vi "niFpgaRegisterEmulation.vi"(0 "name":string, 1 "in timed loop":bool, 5 "Initial Value":variant[](array[variant]), 7 "data in":i32, 9 "write":bool, 11 "error in (no error)":errorcluster, 12 "Local? (F)":bool, 13 "Ref In wired (F)":bool) -> (8 "data out":i32, 15 "error out":errorcluster)   [LabVIEW 2017]
uses:
  <instcachedir>/0/niFpgaRegisterEmulationFpgaImpl_443A04883B3343BC9BF1EB853D0E50EA.lvgen/niFpgaRegisterEmulationFpgaImpl_443A04883B3343BC9BF1EB853D0E50EA_000.vi
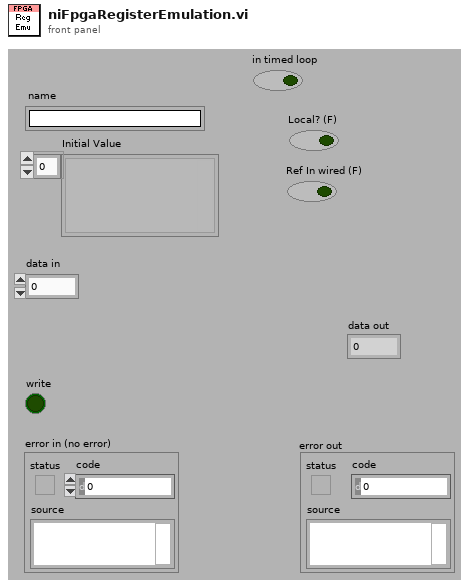
[diagram p1: front panel]
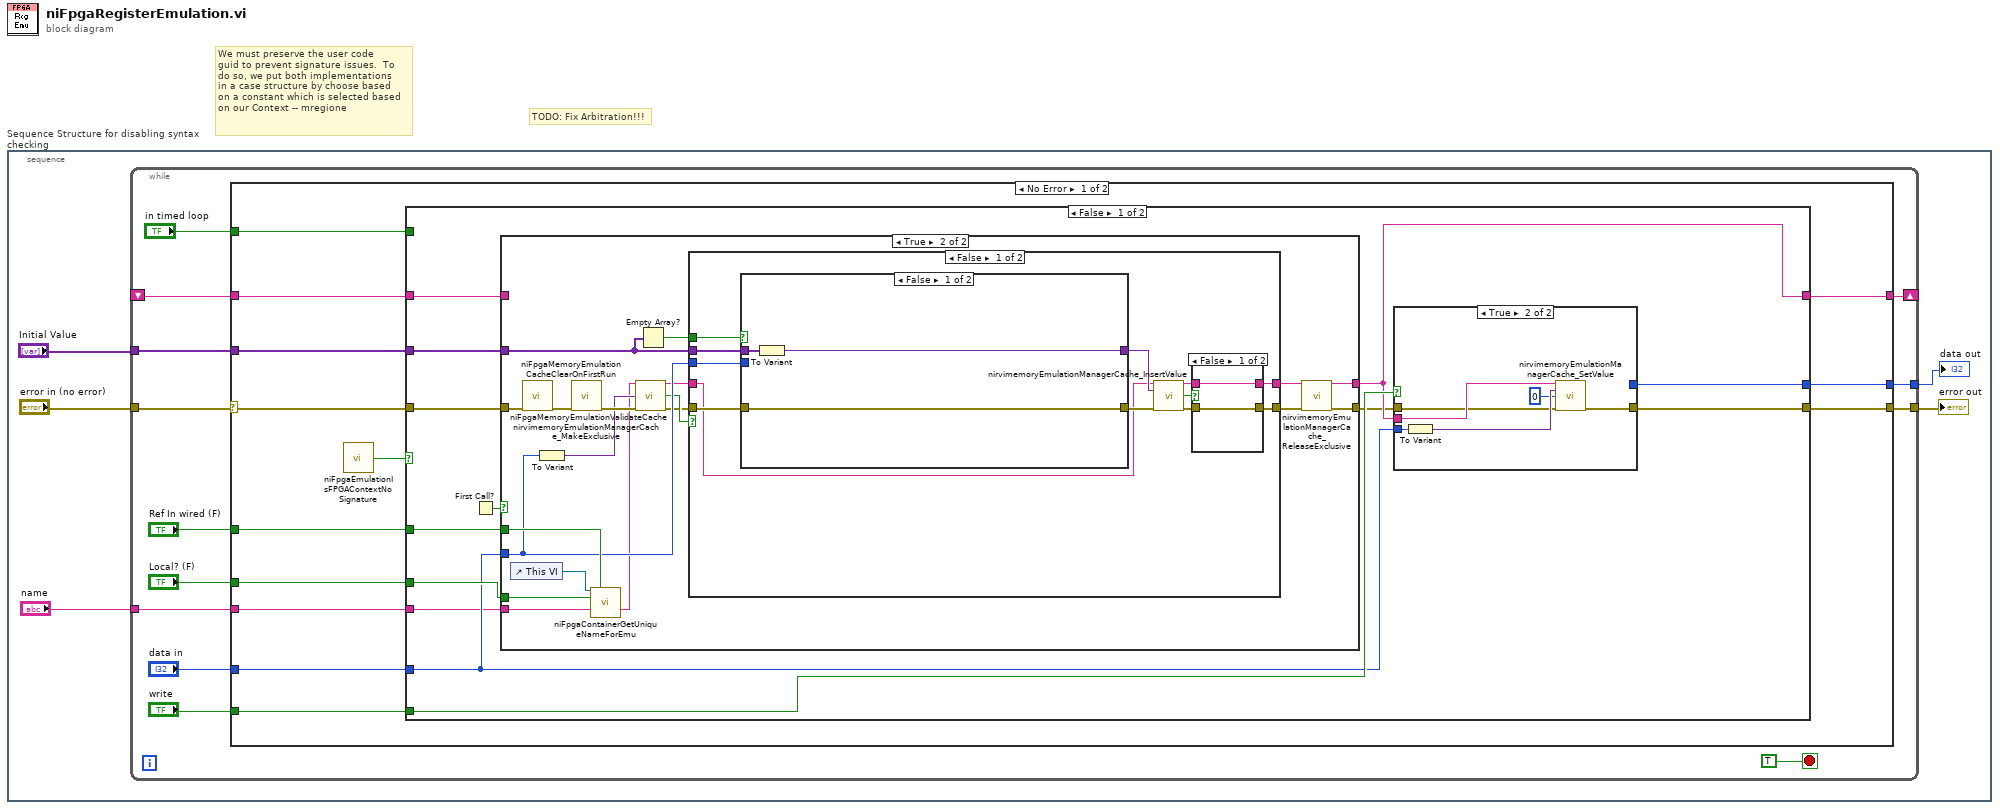
[diagram p0: block diagram]
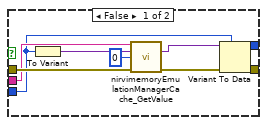
[diagram p2: hidden frame]
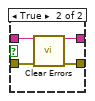
[diagram p4: hidden frame]
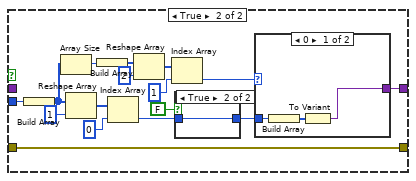
[diagram p5: hidden frame]
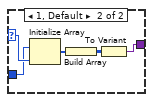
[diagram p6: hidden frame]
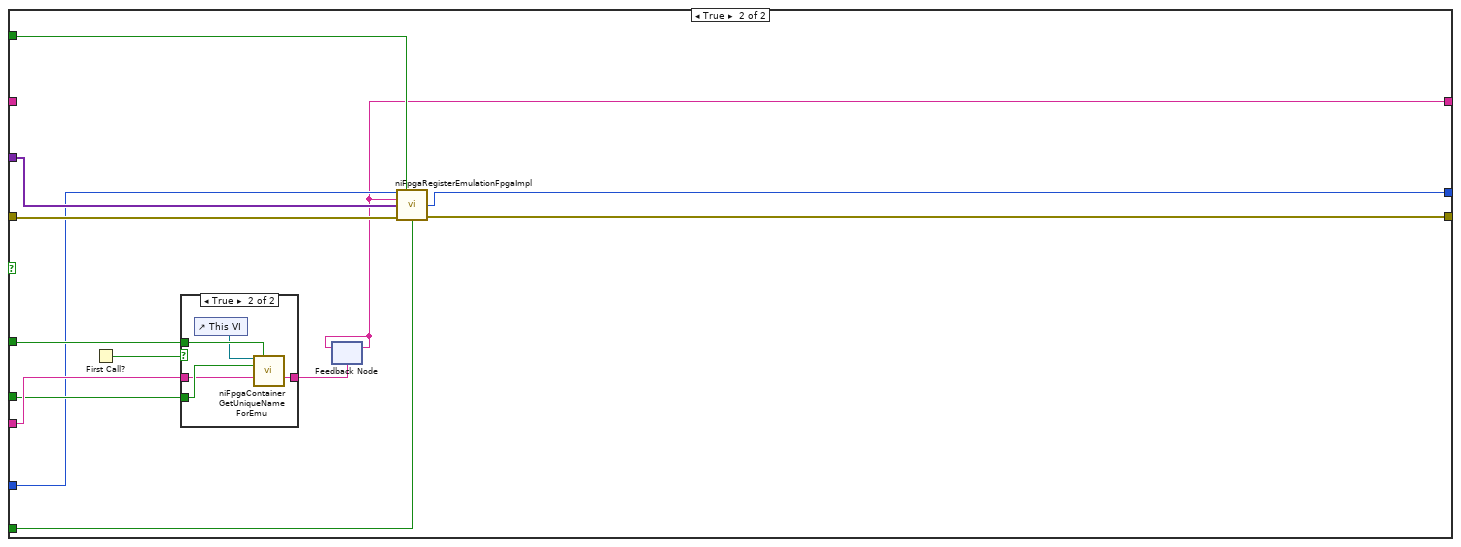
[diagram p9: hidden frame]
diagram:
  # "We must preserve the user code\nguid to prevent signature issues.  To\ndo so, we put both implementations\nin a case structure by choose based\non a constant which is selected based\non our Context -- mregione"
  # "TODO: Fix Arbitration!!!"
  n1 = stacked-sequence "Sequence Structure for disabling syntax checking" {
    frame #0 {
      n2 = while {
        tunnel: [w17] -> w5
        tunnel: "error in (no error)" -> [w15]
        tunnel: "Initial Value" -> [w11]
        shift-right: [w8] -> _
        shift-left: _ -> [w9]
        tunnel: [w7] -> w3
        tunnel: "name" -> [w6]
        stop <- TRUE stop-if-true
        n3 = case shown="No Error" w15 {
          selector: w15 -> [w31 w148]
          tunnel: w11 -> [w28 _]
          tunnel: [w25 w148] -> w17
          tunnel: "data in" -> [w23 w146]
          tunnel: "write" -> [w27 _]
          tunnel: "Ref In wired (F)" -> [w30 _]
          tunnel: "Local? (F)" -> [w29 _]
          tunnel: "in timed loop" -> [w26 _]
          tunnel: w9 -> [w21 w147]
          tunnel: [w20 w147] -> w8
          tunnel: [w24 w146] -> w7
          tunnel: w6 -> [w22 _]
          frame No Error {
            n4 = call <vilib>:"niFpgaEmulationIsFPGAContextNoSignature.vi"() -> ("Is Fpga Context?"=w19:bool)  [unwired: 15 in]
            n5 = case shown="False" w19 {
              tunnel: w31 -> [w44 w134]
              tunnel: w30 -> [w43 w135]
              tunnel: w29 -> [w42 w136]
              tunnel: w28 -> [w41 w132]
              tunnel: w27 -> [w40 w133]
              tunnel: w26 -> [_ w138]
              tunnel: [w39 w128] -> w25
              tunnel: [w38 w129] -> w24
              tunnel: w23 -> [w37 w131]
              tunnel: w22 -> [w36 w137]
              tunnel: w21 -> [w35 _]
              tunnel: [w34 w130] -> w20
              frame False {
                n6 = First Call?() -> (First Call?: T/F=w32:bool)
                n7 = case shown="True" w32 {
                  tunnel: [w61 w64] -> w33
                  tunnel: w44 -> [w61 w63]
                  tunnel: w41 -> [_ w79]
                  tunnel: w37 -> [_ w73]
                  tunnel: w43 -> [_ w77]
                  tunnel: w42 -> [_ w76]
                  tunnel: w36 -> [_ w75]
                  tunnel: [w60 w65] -> w34
                  tunnel: w35 -> [w60 _]
                  frame False {
                  }
                  frame True {
                    n8 = control-ref of="This VI"() -> (w78:refnum<vi>)
                    n9 = call <vilib>:"niFpgaMemoryEmulationCacheClearOnFirstRun.vi"("error in"=w63) -> ("error out"=w62:errorcluster)  [unwired: 13 in, 1 out]
                    n10 = To Variant(anything=w73) -> (Variant=w72:variant)
                    n11 = call <vilib>:"nirvimemoryEmulationManagerCache_MakeExclusive.vi"("error in"=w62) -> ("error out"=w74:errorcluster)  [unwired: 13 in, 1 out]
                    n12 = call <vilib>:"niFpgaContainerGetUniqueNameForEmu.vi"("parent VI"=w78, "ref in wired"=w77, "local"=w76, "name in"=w75) -> ("name out"=w71:string)  [unwired: 11 in]
                    n13 = call <vilib>:"niFpgaMemoryEmulationValidateCache.vi"("key"=w71, "Data In"=w72, "error in"=w74) -> ("key (dup)"=w68:string, "found?"=w70:bool, "error out"=w69:errorcluster)  [unwired: 10 in]
                    n14 = Empty Array?(array=w79) -> (empty?=w80:bool)
                    n15 = case shown="False" w70 {
                      tunnel: w80 -> [w92 _]
                      tunnel: w79 -> [w91 _]
                      tunnel: [w86 w127] -> w67
                      tunnel: w73 -> [w84 _]
                      tunnel: w69 -> [w83 w127]
                      tunnel: w68 -> [w82 w126]
                      tunnel: [w81 w126] -> w66
                      frame False {
                        n16 = case shown="False" w92 {
                          tunnel: w91 -> [w100 _]
                          tunnel: [w99 w102] -> w90
                          tunnel: w84 -> [_ w116]
                          tunnel: w83 -> [w98 w101]
                          tunnel: [w98 w101] -> w87
                          frame False {
                            n17 = To Variant(anything=w100) -> (Variant=w99:variant)
                          }
                          frame True {
                            n18 = Build Array(w116) -> (w115:i32[])
                            n19 = Array Size(array=w115) -> (size(s)=w111:i32)
                            n20 = Reshape Array(w115, 1 ("dimension size")) -> (w113:i32[])
                            n21 = Build Array(w111) -> (w107:i32[])
                            n22 = Index Array(array=w113, index=0) -> (element=w106:i32)
                            n23 = Reshape Array(w107, 2 ("dimension size")) -> (w108:i32[])
                            n24 = Index Array(array=w108, index=1) -> (element=w104:i32)
                            n25 = case shown="True" FALSE {
                              tunnel: w106 -> [_ w125]
                              tunnel: [_ w125] -> w103
                              frame False {
                              }
                              frame True {
                              }
                            }
                            n26 = case shown="0" w104 {
                              selector: w104 -> [_ w124]
                              tunnel: w103 -> [w119 w123]
                              tunnel: [w117 w120] -> w102
                              frame 0 {
                                n27 = Build Array(w119) -> (w118:i32[])
                                n28 = To Variant(anything=w118) -> (Variant=w117:variant)
                              }
                              frame 1, Default {
                                n29 = Initialize Array(w123, w124) -> (w122:i32[])
                                n30 = Build Array(w122) -> (w121:i32[][])
                                n31 = To Variant(anything=w121) -> (Variant=w120:variant)
                              }
                            }
                          }
                        }
                        n32 = call <vilib>:"nirvimemoryEmulationManagerCache_InsertValue.vi"("Key"=w82, "Value"=w90, "error in (no error)"=w87) -> ("Key"=w85:string, "Found"=w89:bool, "error out"=w88:errorcluster)  [unwired: 1 in, 9 out]
                        n33 = case shown="False" w89 {
                          tunnel: w88 -> [w94 w96]
                          tunnel: [w94 w95] -> w86
                          tunnel: [w93 w97] -> w81
                          tunnel: w85 -> [w93 w97]
                          frame False {
                          }
                          frame True {
                            n34 = call <vilib>:"Clear Errors.vi"("error in (no error)"=w96) -> ("error out"=w95:errorcluster)  [unwired: 1 in, 5 out]
                          }
                        }
                      }
                      frame True {
                      }
                    }
                    n35 = call <vilib>:"nirvimemoryEmulationManagerCache_ReleaseExclusive.vi"("Key"=w66, "error in"=w67) -> ("Key (dup)"=w65:string, "error out"=w64:errorcluster)  [unwired: 12 in]
                  }
                }
                n36 = case shown="True" w40 {
                  tunnel: w37 -> [w46 w59]
                  tunnel: w33 -> [w51 w56]
                  tunnel: w34 -> [w50 w57]
                  tunnel: [w48 w55] -> w39
                  tunnel: [w47 _] -> w38
                  frame False {
                    n37 = To Variant(anything=w46) -> (Variant=w53:variant)
                    n38 = call <vilib>:"nirvimemoryEmulationManagerCache_GetValue.vi"("Key"=w50, "Value"=w53, "Address"=0, "error in (no error)"=w51) -> ("Value"=w45:variant, "error out"=w49:errorcluster)  [unwired: 10 out]
                    n39 = Variant To Data(error in=w49, type=w46, Variant=w45) -> (data=w47:i32, error out=w48:errorcluster)
                  }
                  frame True {
                    n40 = To Variant(anything=w59) -> (Variant=w58:variant)
                    n41 = call <vilib>:"nirvimemoryEmulationManagerCache_SetValue.vi"("Key"=w57, "Value"=w58, "Address"=0, "error in (no error)"=w56) -> ("error out"=w55:errorcluster)  [unwired: 11 out]
                  }
                }
              }
              frame True {
                n42 = First Call?() -> (First Call?: T/F=w140:bool)
                n43 = case shown="True" w140 {
                  tunnel: w136 -> [_ w145]
                  tunnel: w135 -> [_ w144]
                  tunnel: [_ w142] -> w139
                  tunnel: w137 -> [_ w141]
                  frame False {
                  }
                  frame True {
                    n44 = control-ref of="This VI"() -> (w143:refnum<vi>)
                    n45 = call <vilib>:"niFpgaContainerGetUniqueNameForEmu.vi"("parent VI"=w143, "ref in wired"=w144, "local"=w145, "name in"=w141) -> ("name out"=w142:string)  [unwired: 11 in]
                  }
                }
                n46 = feedback #1(w139) -> (w130:string)
                n47 = feedback-in #1(w130) -> ()
                n48 = call-generic <vilib>:"niFpgaRegisterEmulationFpgaImpl.vi"("data in"=w131, "In Sctl?"=w138, "name"=w130, "Initial Value"=w132, "error in (no error)"=w134, "Write?"=w133) -> ("data out"=w129:i32, "error out"=w128:errorcluster)  [unwired: 8 in]
              }
            }
          }
          frame Error {
          }
        }
      }
      "error out" <- w5
      "data out" <- w3
    }
  }
